vi "Insight_RW_Sweep_By_Pts_Rate_Step.vi"(6 "Timeout, sec":u32=3, 7 "Sweep Parameters":T1={"Num Points"=2000, "Rate (kHz)"=100.0, "Opt. Freq. Step (GHz)"=0.0, "Min WL (nm)"=1520.0, "Max WL (nm)"=1570.0, "Intersweep Delay (ns)"=100.0, "Total Pts Increment"=4, "Power (mW)"=10.0, "Power Profile"=enum."FLAT", "Edge Roll-off (dB)"=10.0, "WL Sweep Direction?"=enum."Increase"}, 8 "error in (no error)":errorcluster, 9 "Mode (Read / Write)":enum8{"Write", "Read"}(ring), 10 "Sweep Cal Type":T3(radio), 11 "telnet connection":T4) -> (0 "error out":errorcluster, 2 "response data":string, 3 "telnet connection out":T4)   [LabVIEW 2015]
doc: "Insight Photonic Solutions\n\nThis VI configures the sweep of the akinetic laser to prioritize sweeping by Points, by Sweep Rate or by Optical Frequency Step. Additional parameters configured for the sweep are minimum wavelength, maximum wavelength and duty cycle.\n\nTo implement the requested sweep configuration, please send the command \":CALibrate:SWEep\" via the \"Insight_RW_Sweep_Calibrate.vi\"\n\nINPUTS\n\ntelnet connection - specifies the Telnet connection to the laser\nMode (Read/Write) - defines if the command is a read or write of the configuration\nSweep Cal Type - defines if the configuration is \"Sweep by Number\", \"Sweep by Rate\" or \"Sweep by Step\".\nSweep Parameters - defines the sweep paramaters to be configured. This cluster also contains the power, power profile and roll-off commands, but these are not configured in this VI.\nTimeout, sec - the Telnet communication timeout allowed\nerror in - LabView's error cluster, used to track errors and enforce sequentiality in your code\n\nOUTPUTS\n\ntelnet connection out - passes out the Telnet connection reference\nresponse data - the string returned by the laser in response to a read or write of sweep configuration\nerror out - LabView's error cluster, used to track errors and enforce sequentiality in your code\n\nREVISION HISTORY\nver 3.5 - original release"
uses:
  Telnet Session.ctl
  Sweep Parameters.ctl
  Power_Profiles.ctl
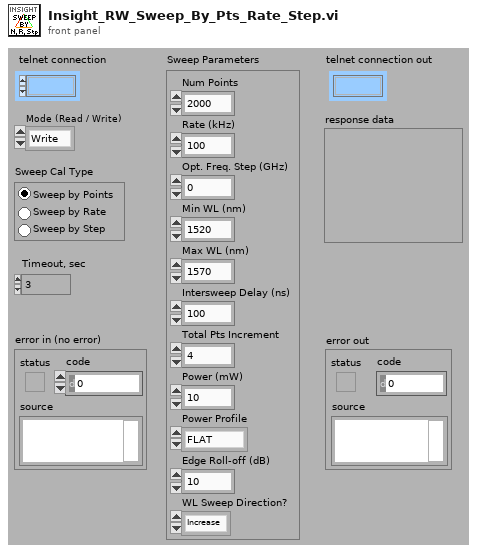
[diagram p1: front panel]
types:
  T1 = typedef "Sweep Parameters.ctl" = cluster{"Num Points":u32, "Rate (kHz)":dbl, "Opt. Freq. Step (GHz)":dbl, "Min WL (nm)":dbl, "Max WL (nm)":dbl, "Intersweep Delay (ns)":dbl, "Total Pts Increment":u32, "Power (mW)":dbl, "Power Profile":T2, "Edge Roll-off (dB)":dbl, "WL Sweep Direction?":enum16{"Increase", "Decrease", "Bidirectional_Increase", "Bidirectional_Decrease"}}
  T2 = typedef "Power_Profiles.ctl" = enum16{"FLAT", "GAUSsian", "CUSTom"}
  T3 = enum32{"Sweep by Points", "Sweep by Rate", "Sweep by Step"}
  T4 = typedef "Telnet Session.ctl" = refnum<k1>
  T5 = enum16{"Increase", "Decrease", "Bidirectional_Increase", "Bidirectional_Decrease"}
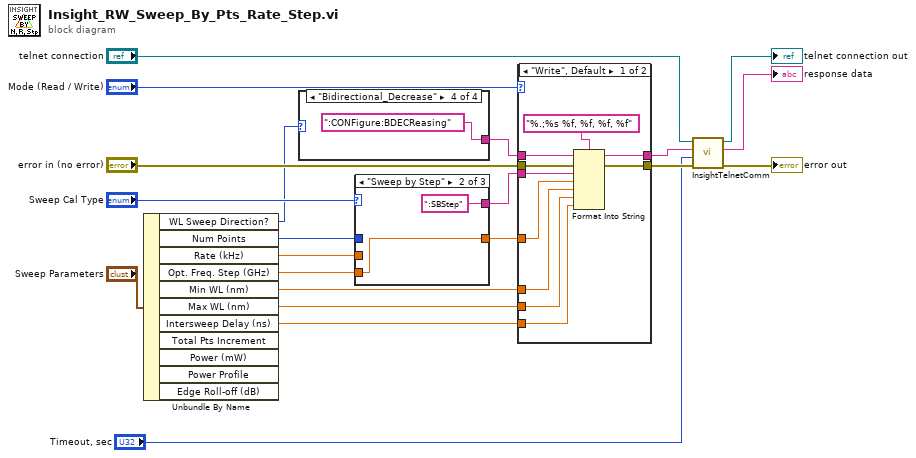
[diagram p0: block diagram]
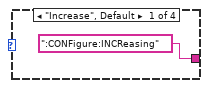
[diagram p2: hidden frame]
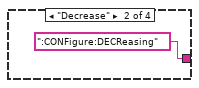
[diagram p3: hidden frame]
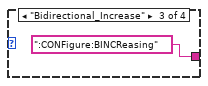
[diagram p4: hidden frame]
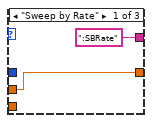
[diagram p5: hidden frame]
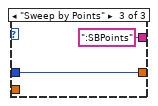
[diagram p6: hidden frame]
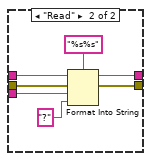
[diagram p7: hidden frame]
diagram:
  n1 = Unbundle By Name("Sweep Parameters") -> ("WL Sweep Direction?"=w2:T5, "Num Points"=w10:u32, "Rate (kHz)"=w9:dbl, "Opt. Freq. Step (GHz)"=w8:dbl, "Min WL (nm)"=w4:dbl, "Max WL (nm)"=w5:dbl, "Intersweep Delay (ns)"=w6:dbl)  [unwired: 4 out]
  n2 = case shown="\"Bidirectional_Decrease\"" w2 {
    tunnel: [":CONFigure:INCReasing" ":CONFigure:DECReasing" ":CONFigure:BINCReasing" ":CONFigure:BDECReasing"] -> w3
    frame "Increase", Default {
    }
    frame "Decrease" {
    }
    frame "Bidirectional_Increase" {
    }
    frame "Bidirectional_Decrease" {
    }
  }
  n3 = case shown="\"Sweep by Step\"" "Sweep Cal Type" {
    tunnel: [":SBRate" ":SBStep" ":SBPoints"] -> w13
    tunnel: w10 -> [_ _ w30]
    tunnel: w9 -> [w26 _ _]
    tunnel: w8 -> [_ w28 _]
    tunnel: [w26 w28 w30] -> w7
    frame "Sweep by Rate" {
    }
    frame "Sweep by Step" {
    }
    frame "Sweep by Points" {
    }
  }
  n4 = case shown="\"Write\", Default" "Mode (Read / Write)" {
    tunnel: [w41 w45] -> w20
    tunnel: "error in (no error)" -> [w40 w44]
    tunnel: w3 -> [w39 w47]
    tunnel: [w37 w46] -> w19
    tunnel: w13 -> [w36 w43]
    tunnel: w7 -> [w35 _]
    tunnel: w4 -> [w34 _]
    tunnel: w5 -> [w33 _]
    tunnel: w6 -> [w32 _]
    frame "Write", Default {
      n5 = Format Into String(format string="%.;%s %f, %f, %f, %f", initial string=w39, error in=w40, w36, w35, w34, w33, w32) -> (resulting string=w37:string, error out=w41:errorcluster)
    }
    frame "Read" {
      n6 = Format Into String(format string="%s%s", initial string=w47, error in=w44, w43, "?" ("input 1")) -> (resulting string=w46:string, error out=w45:errorcluster)
    }
  }
  n7 = call "InsightTelnetComm.vi"("error in"=w20, "Timeout, sec"="Timeout, sec", "write buffer (\"\")"=w19, "telnet connection"="telnet connection") -> ("error out"=→"error out":errorcluster, "response data"=→"response data":string, "telnet  connection out"=→"telnet connection out":T4)  [unwired: 3 in]
